vi "TSM Get TIB Settings.vi"(0 "TSM context In":T1, 11 "error in (no error)":errorcluster) -> (4 "TSM context Out":T1, 6 "External Resistance (Ohm)":dbl, 15 "error out":errorcluster)   [LabVIEW 2020]
uses:
  <vilib>/NI_TestStand_SemiconductorModule/NI_TestStand_Semiconductor_Module.lvlibp/PinMap/General/SemiconductorModuleContext.ctl
  <vilib>/NI_TestStand_SemiconductorModule/NI_TestStand_Semiconductor_Module.lvlibp/PinMap/Specs/NamespacedSymbolsToValues.vi
  <vilib>/NI_TestStand_SemiconductorModule/NI_TestStand_Semiconductor_Module.lvlibp
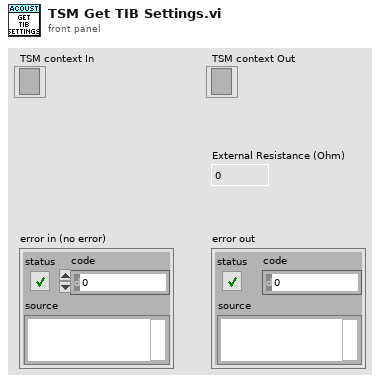
[diagram p1: front panel]
types:
  T1 = typedef "NI_TestStand_Semiconductor_Module.lvlibp/SemiconductorModuleContext.ctl" = refnum<k7>
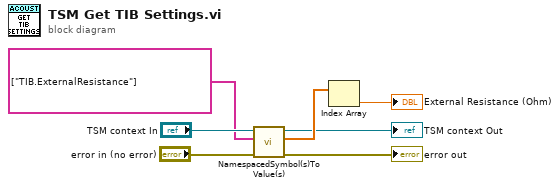
[diagram p0: block diagram]
diagram:
  n1 = call-poly <vilib>:"NamespacedSymbol(s)ToValue(s).vi"("error in (no error)"="error in (no error)", "Symbols"=tag[] ["TIB.ExternalResistance"], "Semiconductor Module Context"="TSM context In") -> ("error out"=→"error out":errorcluster, "Values"=w4:dbl[], "Semiconductor Module Context Out"=→"TSM context Out":T1)  [unwired: 6 in]
  n2 = Index Array(array=w4) -> (element=→"External Resistance (Ohm)":dbl)  [unwired: 1 in]
